vi "Read PID controller configuration.vi"(8 "error in (no error)":errorcluster, 11 "PID Controller in":refnum<class "PID Controller.lvclass">) -> (0 "error out":errorcluster, 2 "Configuration":T1, 3 "PID Controller out":refnum<class "PID Controller.lvclass">)   [LabVIEW 2018, in "PID Controller.lvclass"]
uses:
  PID Controller.lvclass
  C:/github/LabActor/Template Module/Template Module.lvclass
  PID Controller Configuration.ctl
  Template Module/Template Module.lvclass/Template Module.ctl
  Template Module/Read Configuration.vi
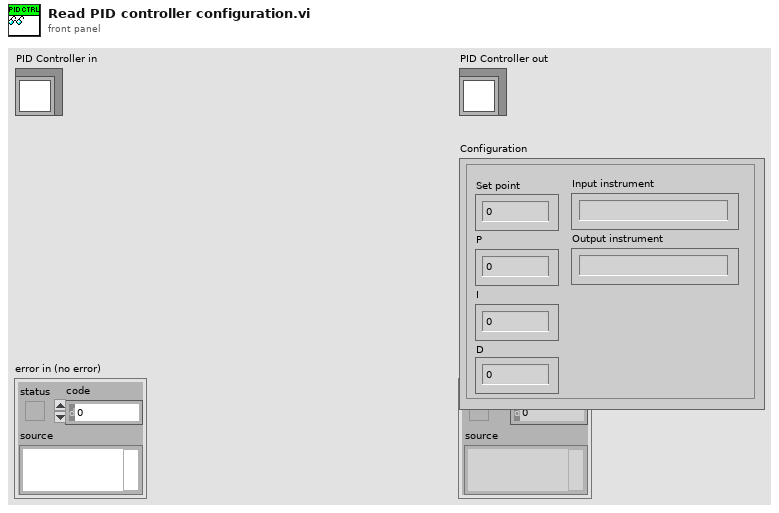
[diagram p1: front panel]
types:
  T1 = typedef "PID Controller Configuration.ctl" = cluster{"P":dbl, "I":dbl, "D":dbl, "Set point":dbl, "Input instrument":string, "Output instrument":string}
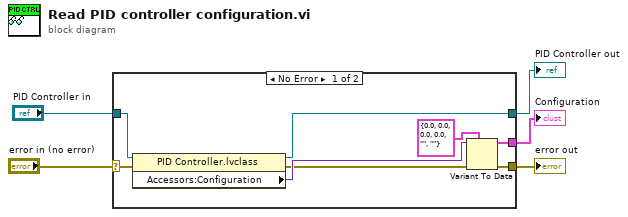
[diagram p0: block diagram]
diagram:
  n1 = case shown="No Error" "error in (no error)" {
    selector: "error in (no error)" -> [w13 w14]
    tunnel: [w7 w14] -> w4
    tunnel: [w11 w15] -> w2
    tunnel: "PID Controller in" -> [w12 w15]
    tunnel: [w8 _] -> w1
    frame No Error {
      n2 = property class="PID Controller.lvclass"(reference=w12, error in=w13) -> (reference out=w11:refnum<class "PID Controller.lvclass">, error out=w6:errorcluster, "Accessors:Configuration"=w9:variant)
      n3 = Variant To Data(error in=w6, type=T1 {"P"=0.0, "I"=0.0, "D"=0.0, "Set point"=0.0, "Input instrument"="", "Output instrument"=""} ("Configuration"), Variant=w9) -> (data=w8:T1, error out=w7:errorcluster)
    }
    frame Error {
    }
  }
  "error out" <- w4
  "PID Controller out" <- w2
  "Configuration" <- w1
